vi "CO2FeedbackControl.vi"() -> ()   [LabVIEW 2020]
uses:
  <vilib>/Utility/file.llb/Write Delimited Spreadsheet (DBL).vi
  <vilib>/Analysis/NI_AALPro.lvlib
panel:
  in  "N":i32=30
  in  "file path (dialog if empty) 3":path=path "C:/Users/user/Desktop/CO2_Laptop/Data/data"
  in  "format (%.3f) 2":string="%.5f"
  in  "Save File 2":bool
  in  "file path (dialog if empty) 4":path=path "C:/Users/user/Desktop/CO2_Laptop/Data/210528"
  out "appended path 3":path=path "C:/Users/user/Desktop/CO2_Laptop/Data/210528/81757"
  in  "Save All":bool
  in  "Saving File Time(Sec)":dbl=60.0
  in  "Safty Check":bool=TRUE
  out "> Thres 2":bool
  in  "Slope Set":dbl=300.0
  out "Time Number":u32=81757
  out "String":string="081757\r\n"
  in  "Save Background":bool
  out "> Thres":bool
  in  "stop":bool
  in  "Integration Time(ms)":i32=85
  in  "Average Times":i32=4
  in  "Wait Time":u32=120
  in  "UV450 Set":sgl=383500.0
  in  "Rate (ml/min)":dbl=0.0045
  out "Dose or Not":i32
  in  "Pump Time":u32=1000
  in  "Connect the Pump":bool=TRUE
  in  "Setting Tab":T1(tab)
  out "On/Off":i32(graph)
  out "Derative Signal":dbl(graph)=-0.9345383759733037
  out "FADH":sgl(graph)=81856.375
  out "?":sgl=81856.375
  out "?":sgl=1683298.0
  out "UV300":sgl=1683274.0
  out "Fc+":sgl(graph)=1683274.0
  out "NADH":sgl(graph)=1683298.0
  out "U300 Slope":dbl=-0.9345383759733037
  in  "Initial Number":dbl
  in  "Initial Wavelength 2":dbl=275.0
  out "Index 2":dbl=125.0
  in  "Final Wavelength":dbl=620.0
  out "Index 3":dbl=576.0
  out "subarray 2":sgl[](array[numeric])=[332.8669, 333.6288, 334.39072, 335.15262, 335.9145, 336.67633, 337.43814, 338.19995, 338.96173, 339.72348, 340.4852, 341.24692, 342.0086, 342.77026, 343.53192, 344.29355, 345.05515, 345.8167, 346.57825, 347.33978, 348.10126, 348.86273, 349.6242, 350.38562, 351.147, 351.9084]
  out "subarray":sgl[](array[numeric])=[446.05103, 446.80762, 447.56418, 448.32068, 449.07715, 449.83356, 450.5899, 451.34622, 452.1025, 452.8587, 453.6149, 454.371, 455.12708, 455.8831, 456.63907, 457.395, 458.15088, 458.9067, 459.66248, 460.4182, 461.1739, 461.92953, 462.68512, 463.44064, 464.19614, 464.95157]
  in  "index":i32=350
  in  "length 3":i32=26
  in  "index 2":i32=201
  out "Background":sgl[](graph)=[172.21637, 178.6098, 190.38326, 201.36111, 203.4611, 197.77924, 190.34503, 202.32442, 224.52594, 247.76048, 288.25705, 329.7657, 369.02264, 416.01242, 476.80292, 575.00824, 737.26373, 961.8769, 1266.476, 1647.3512, 2141.3354, 2791.3042, 3647.9653, 4759.415, 6167.531, 7863.0625, 9861.403, 12171.496, 14761.8125, 17573.484, 20526.473, 23478.443, 26351.168, 29083.691, 31614.525, 33886.91, 35870.95, 37502.207, 38754.105, 39600.734, 40049.812, 40105.33, 39828.324, 39231.23, 38360.957, 37355.445, 36104.72, 34783.223, 33399.88, 31985.346, 30560.78, 29142.305, 27749.982, 26391.615, 25085.277, 23821.594, 22594.584, 21429.28, 20331.139, 19246.326, 18235.92, 17305.72, 16387.797, 15554.422, 14779.023, 14065.231, 13400.149, 12777.7295, 12199.317, 11662.219, 11158.4375, 10707.728, 10302.769, 9948.339, 9619.979, 9311.22, 9019.734, 8746.263, 8497.579, 8287.871, 8119.847, 7988.0596, 7882.8696, 7806.2563, 7740.983, 7700.281, 7682.2935, 7665.853, 7679.71, 7699.8457, 7742.342, 7819.9507, 7932.1553, 8081.9766, 8245.204, 8436.354, 8637.018, 8861.075, 9118.328, 9391.317, 9705.655, 10059.682, 10457.724, 10911.704, 11425.339, 11995.643, 12610.294, 13264.511, 13950.56, 14684.349, 15458.021, 16279.438, 17157.658, 18103.229, 19112.172, 20207.807, 21388.975, 22639.855, 23991.432, 25457.422, 27022.8, 28664.277, 30323.066, 32030.035, 33610.438, 35245.04, 36934.887, 38771.98, 40825.938, 43076.9, 45512.37, 48168.47, 50984.766, 53626.605, 56118.92, 58950.207, 61775.047, 63773.973, 63949.07, 64084.047, 64178.383, 64184.605, 64149.074, 64052.793, 63915.992, 63918.89, 64040.336, 64118.902, 64116.21, 64092.902, 64052.22, 64033.504, 64038.297, 64028.242, 64027.098, 64060.793, 64076.066, 64126.375, 64043.8, 63250.496, 61768.496, 60734.766, 59729.53, 57698.125, 54165.81, 50176.914, 46149.234, 42733.66, 39790.543, 37493.91, 35500.812, 33451.094, 31229.004, 28788.117, 26540.094, 24475.693, 22718.572, 21113.527, 19627.281, 18206.932, 16862.273, 15712.507, 14730.38, 13751.289, 12770.087, 11858.61, 11046.73, 10340.737, 9747.756, 9237.91, 8805.616, 8444.61, 8120.295, 7834.2686, 7539.886, 7164.0596, 6707.6084, 6190.263, 5689.185, 5312.52, 5098.453, 4977.2, 4910.097, 4891.2104, 4864.877, 4698.309, 4427.4155, 4232.314, 4121.4736, 4006.222, 3878.76, 3771.4011, 3690.84, 3640.2373, 3603.596, 3591.162, 3573.36, 3571.922, 3578.0845, 3617.4995, 3670.426, 3743.4565, 3818.7466, 3857.2388, 3859.1992, 3828.7473, 3787.6472, 3752.0144, 3739.1199, 3729.3882, 3729.4111, 3711.954, 3675.612, 3636.6428, 3600.4456, 3568.309, 3558.572, 3548.6543, 3553.8538, 3585.2307, 3649.1536, 3724.6, 3798.702, 3789.903, 3713.3398, 3570.3772, 3424.1174, 3351.6611, 3369.2878, 3452.262, 3535.7366, 3538.5234, 3437.643, 3262.2917, 3037.4912, 2832.5955, 2661.3347, 2508.405, 2392.6135, 2306.7063, 2273.7944, 2276.2817, 2301.8428, 2296.0056, 2258.3638, 2196.5005, 2115.8386, 2057.6409, 2045.1534, 2070.7346, 2122.393, 2100.536, 2018.3241, 1882.6237, 1799.5573, 1897.3712, 2203.182, 2784.7966, 3397.9448, 3467.0032, 2968.6287, 2293.2832, 1670.7052, 1317.4867, 1272.086, 1250.7498, 1187.051, 1207.0577, 1242.5907, 1185.1292, 1063.2871, 986.917, 961.3804, 934.924, 907.7848, 873.4408, 833.07916, 792.1351, 748.04736, 694.6823, 654.212, 617.8926, 585.5748, 555.31824, 530.2687, 512.13306, 502.65018, 484.0129, 461.54538, 436.27756, 404.15952, 379.0401, 336.2221, 303.73672, 269.4475, 242.80533, 231.45448, 222.27428, 226.29994, 221.17111, 211.7707, 199.02214, 187.00967, 167.50746, 160.57787, 158.06314, 145.95668, 140.2896, 143.32124, 142.59326, 145.61113, 140.5319, 125.95628, 115.798744, 104.68489, 91.8871, 84.10792, 83.73946, 79.02437, 89.39399, 93.75515, 103.549706, 113.17898, 119.95357, 112.730675, 107.5902, 98.01945, 93.53506, 81.586525, 71.61932, 63.659184, 70.39902, 75.41178, 91.91837, 104.64616, 116.470856, 121.41953, 125.59211, 116.32846, 110.59207, 97.97765, 85.71354, 72.04285, 70.710396, 77.94153, 104.69237, 128.20029, 134.88873, 131.4962, 110.10464, 84.07277, 67.67252, 59.044857, 58.778107, 64.593765, 69.131714, 66.15145, 69.076164, 71.793076, 71.89148, 69.14369, 61.262066, 54.19736, 46.46217, 35.316803, 10.673843, 0.65000325, 3.4500182, 21.898348, 51.27786, 87.18853, 101.60523, 93.91958, 76.44091, 50.19149, 32.17609, 34.534836, 40.355633, 55.11234, 64.29569, 72.62746, 80.33474, 80.12523, 75.10533, 67.51369, 49.410484, 36.219204, 26.42124, 36.805626, 43.322285, 58.033817, 65.59648, 68.226845, 64.07072, 62.22196, 56.900043, 44.901432, 42.843807, 33.538353, 31.444857, 31.923042, 27.305967, 28.892494, 34.93258, 44.089443, 56.331985, 72.50936, 71.152855, 65.88946, 58.713154, 44.860325, 35.122955, 25.37532, 20.282688, 20.226677, 29.445103, 47.947227, 68.52041, 90.17749, 103.97235, 99.2943, 81.80186, 61.792732, 48.94577, 34.207508, 40.06172, 48.37855, 54.032833, 64.7118, 79.192184, 89.2192, 95.4683]
  in  "index 3":i32=145
  in  "length":i32=26
  out "subarray 3":sgl[](array[numeric])=[290.1744, 290.93707, 291.6997, 292.46237, 293.225, 293.98764, 294.75027, 295.5129, 296.2755, 297.03812, 297.80072, 298.56332, 299.3259, 300.08847, 300.851, 301.6136, 302.37613, 303.13864, 303.90118, 304.6637, 305.42618, 306.1887, 306.95117, 307.71362, 308.47607, 309.23853]
  out "While Number Now":dbl=60.0
  in  "Wavelength":dbl=455.0
  out "Index":dbl=360.0
  in  "Slope":bool=TRUE
  out "subarray 5":dbl[](array[numeric])=[1683269.0, 1683298.375, 1683359.625, 1683206.625, 1683395.5, 1683321.875, 1683329.125, 1683184.25, 1683210.75, 1683321.25, 1683323.75, 1683204.75, 1683348.5, 1683351.75, 1683382.25, 1683268.0, 1683432.25, 1683458.25, 1683313.375, 1683185.25, 1683231.25, 1683440.875, 1683121.25, 1683666.5, 1683304.0, 1683178.75, 1683377.75, 1683289.5, 1683221.625, 1683048.25]
  out "Array 2":i32[](array[numeric])=[1, 2, 3, 4, 5, 6, 7, 8, 9, 10, 11, 12, 13, 14, 15, 16, 17, 18, 19, 20, 21, 22, 23, 24, 25, 26, 27, 28, 29, 30]
  out "Raw Data Graph 3":cluster{"Lumda":sgl[], "Intensity":sgl[]}(graph)
  out "Trans (Signal >275nm is more stable)":cluster{"Lumda":sgl[], "Intensity":sgl[]}(graph)
  # "Signal Up; More Transparent"
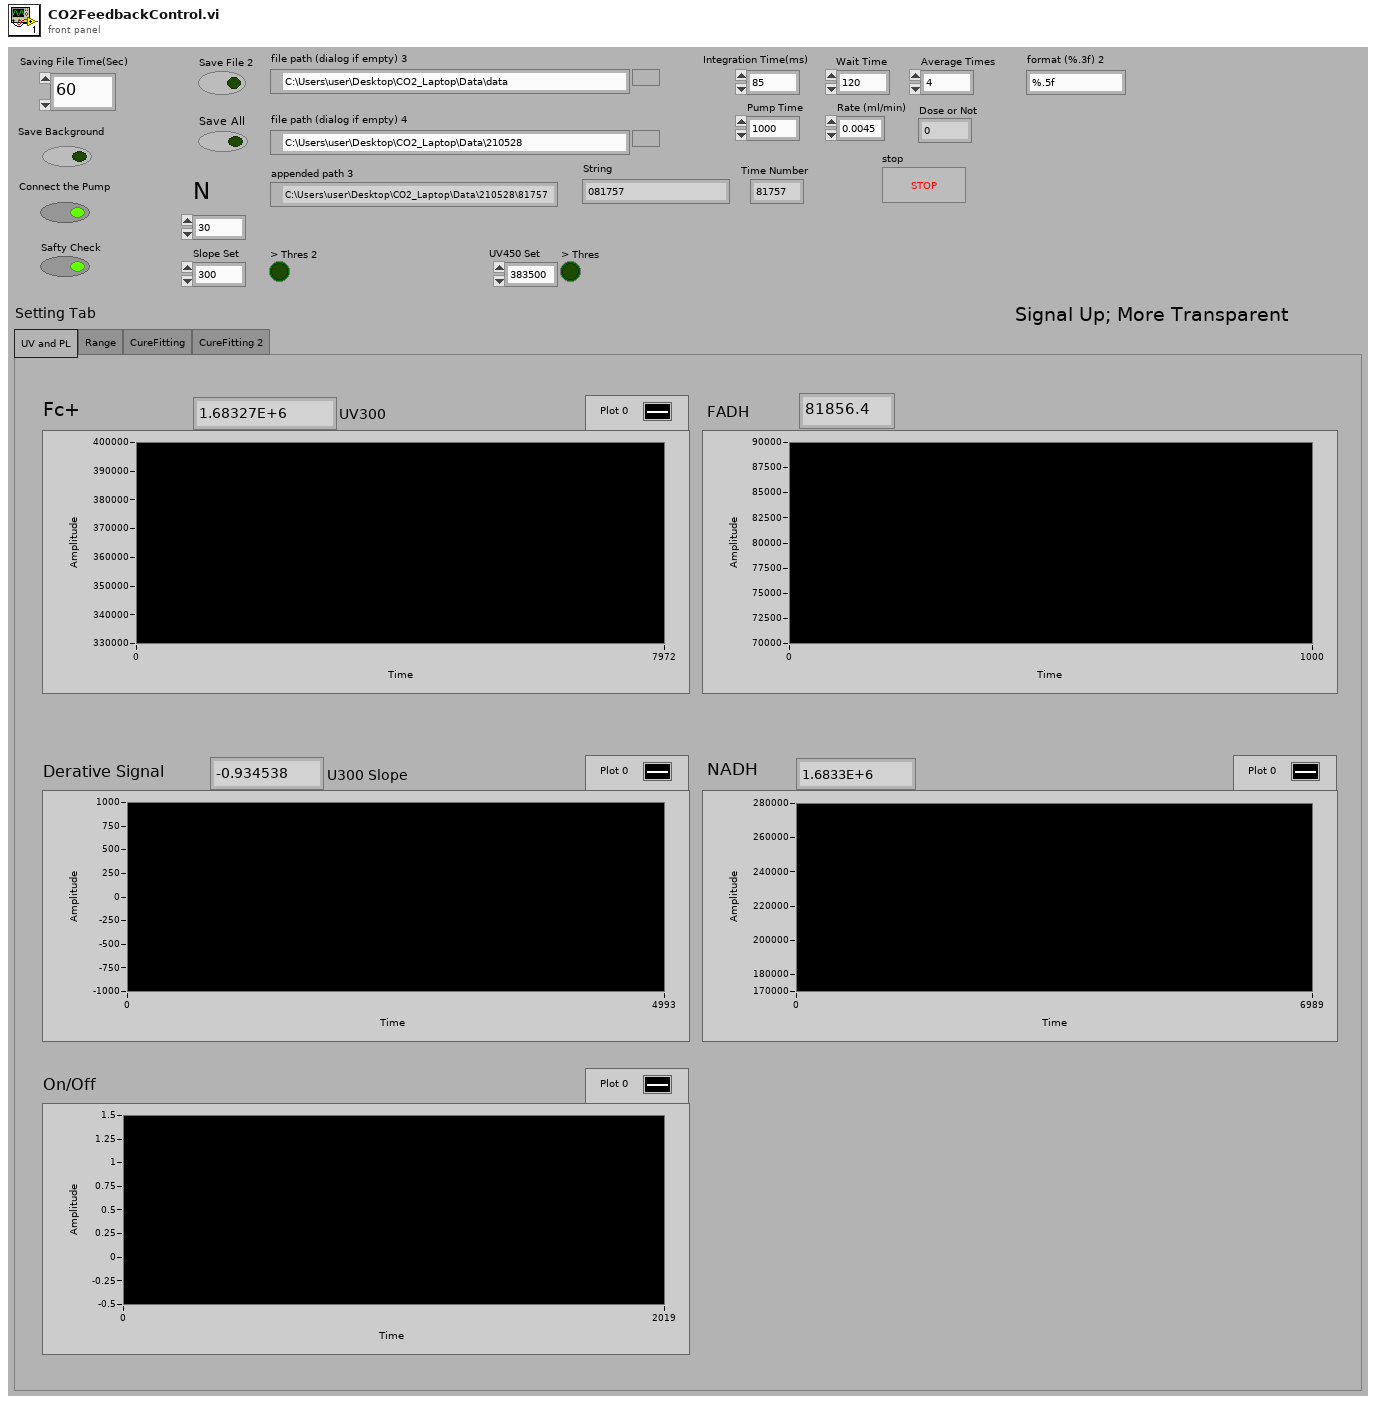
[diagram p1: front panel]
types:
  T1 = enum32{"UV and PL", "Range", "CureFitting", "CureFitting 2"}
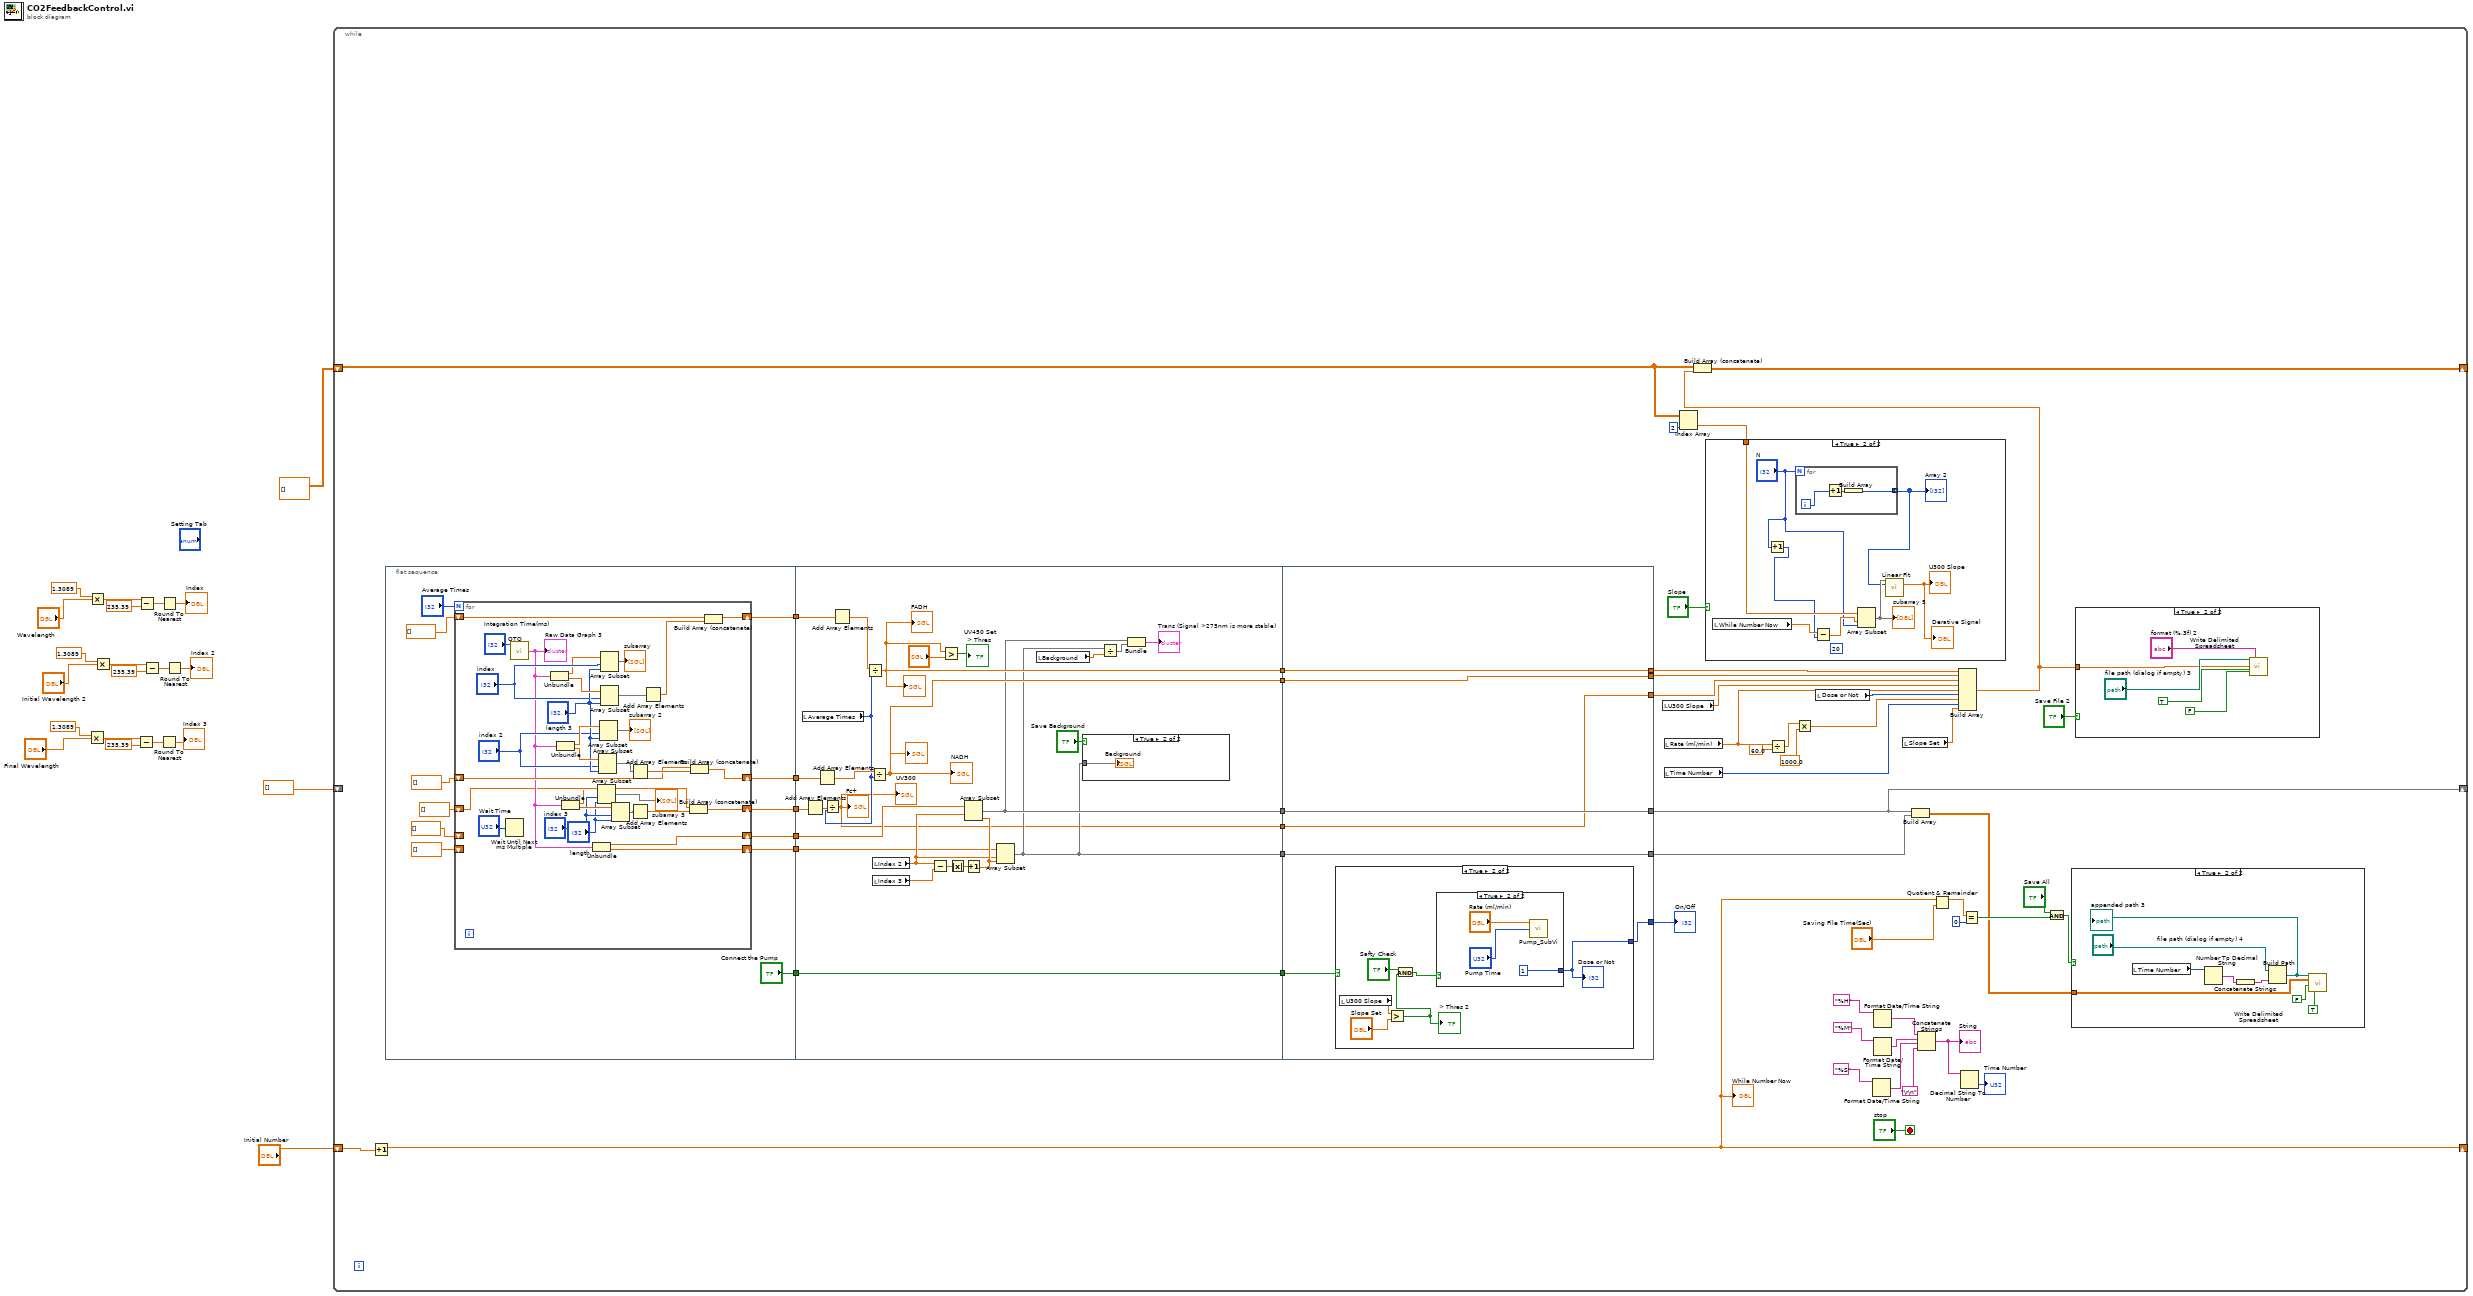
[diagram p0: block diagram]
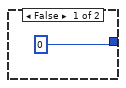
[diagram p6: hidden frame]
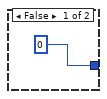
[diagram p7: hidden frame]
diagram:
  n1 = Multiply(x=1.3089, y="Final Wavelength") -> (x*y=w7:dbl)
  n2 = Multiply(x=1.3089, y="Wavelength") -> (x*y=w20:dbl)
  n3 = Multiply(x=1.3089, y="Initial Wavelength 2") -> (x*y=w13:dbl)
  n4 = Subtract(x=w7, y=235.39) -> (x-y=w6:dbl)
  n5 = Subtract(x=w20, y=235.39) -> (x-y=w19:dbl)
  n6 = Subtract(x=w13, y=235.39) -> (x-y=w12:dbl)
  n7 = Round To Nearest(number=w6) -> (nearest integer value=→"Index 3":dbl)
  n8 = Round To Nearest(number=w19) -> (nearest integer value=→"Index":dbl)
  n9 = Round To Nearest(number=w12) -> (nearest integer value=→"Index 2":dbl)
  n10 = while {
    shift-right: [w67] -> _
    shift-left: sgl[][] [] -> [w48]
    shift-right: [w30] -> _
    shift-left: sgl[] [] -> [_]
    shift-right: [w23] -> _
    shift-left: "Initial Number" -> [w49]
    stop <- "stop" stop-if-true
    n11 = Increment(x=w49) -> (x+1=w23:dbl)
    "While Number Now" <- w23
    n12 = flat-sequence {
      tunnel: [w105] -> w73
      tunnel: [w104] -> w72
      tunnel: ["Connect the Pump"] -> w68
      tunnel: [w102] -> w66
      tunnel: [w101] -> w65
      tunnel: [w99] -> w52
      tunnel: w73 -> [w156]
      tunnel: w72 -> [w155]
      tunnel: [w158] -> w71
      tunnel: [w157] -> w70
      tunnel: [w154] -> w69
      tunnel: w68 -> [w154]
      tunnel: w66 -> [w153]
      tunnel: w65 -> [w152]
      tunnel: [w147] -> w63
      tunnel: [w149] -> w62
      tunnel: w52 -> [w145]
      tunnel: [w142] -> w51
      tunnel: [w174] -> w26
      tunnel: [w175] -> w27
      tunnel: w71 -> [w175]
      tunnel: w70 -> [w174]
      tunnel: w69 -> [w173]
      tunnel: [w172] -> w64
      tunnel: w63 -> [w172]
      tunnel: w62 -> [w171]
      tunnel: [w171] -> w30
      tunnel: w51 -> [w170]
      tunnel: [w170] -> w28
      tunnel: [w169] -> w22
      frame #0 {
        n13 = for {
          N: "Average Times" -> [_]
          shift-right: [w135] -> w105
          shift-left: sgl[] [] -> [w134]
          shift-right: [w131] -> w104
          shift-left: sgl[] [] -> [w130]
          shift-right: [w127] -> w101
          shift-left: sgl[] [] ("Intensity") -> [_]
          shift-right: [w126] -> w102
          shift-left: sgl[] [] -> [_]
          shift-right: [w116] -> w99
          shift-left: sgl[] [] -> [w115]
          n14 = Wait Until Next ms Multiple(millisecond multiple="Wait Time") -> ()  [unwired: 1 out]
          n15 = call "OTO.vi"("Integration Time(ms)"="Integration Time(ms)") -> ("Raw Data Graph"=w119:cluster{"Lumda":sgl[], "Intensity":sgl[]})  [unwired: 2 in]
          "Raw Data Graph 3" <- w119
          n16 = Unbundle(w119) -> ("Lumda"=w123:sgl[], "Intensity"=w140:sgl[])
          n17 = Unbundle(w119) -> ("Lumda"=w139:sgl[], "Intensity"=w138:sgl[])
          n18 = Unbundle(w119) -> ("Lumda"=w113:sgl[], "Intensity"=w118:sgl[])
          n19 = Unbundle(w119) -> ("Lumda"=w126:sgl[], "Intensity"=w127:sgl[])
          n20 = Array Subset(array=w113, index="index 3", length="length") -> (→"subarray 3":sgl[])
          n21 = Array Subset(array=w138, index="index 2", length="length 3") -> (w128:sgl[])
          n22 = Array Subset(array=w139, index="index 2", length="length 3") -> (→"subarray 2":sgl[])
          n23 = Array Subset(array=w140, index="index", length="length 3") -> (w133:sgl[])
          n24 = Array Subset(array=w123, index="index", length="length 3") -> (→"subarray":sgl[])
          n25 = Array Subset(array=w118, index="index 3", length="length") -> (w120:sgl[])
          n26 = Add Array Elements(numeric array=w128) -> (sum=w132:sgl)
          n27 = Add Array Elements(numeric array=w120) -> (sum=w117:sgl)
          n28 = Add Array Elements(numeric array=w133) -> (sum=w129:sgl)
          n29 = Build Array (concatenate)(w115, w117) -> (w116:sgl[])
          n30 = Build Array (concatenate)(w130, w132) -> (w131:sgl[])
          n31 = Build Array (concatenate)(w134, w129) -> (w135:sgl[])
        }
      }
      frame #1 {
        n32 = local read "Average Times"() -> (w143:i32)
        n33 = Add Array Elements(numeric array=w145) -> (sum=w144:sgl)
        n34 = Add Array Elements(numeric array=w155) -> (sum=w159:sgl)
        n35 = Divide(x=w144, y=w143) -> (x/y=w142:sgl)
        "Fc+" <- w142
        "UV300" <- w142
        n36 = Add Array Elements(numeric array=w156) -> (sum=w160:sgl)
        n37 = Divide(x=w160, y=w143) -> (x/y=w157:sgl)
        "FADH" <- w157
        "?" <- w157
        n38 = Divide(x=w159, y=w143) -> (x/y=w158:sgl)
        "NADH" <- w158
        "?" <- w158
        n39 = local read "Index 2"() -> (w166:dbl)
        n40 = local read "Index 3"() -> (w163:dbl)
        n41 = Subtract(x=w166, y=w163) -> (x-y=w162:dbl)
        n42 = Greater?(x=w157, y="UV450 Set") -> (0:→"> Thres":bool)
        n43 = Absolute Value(x=w162) -> (abs(x)=w161:dbl)
        n44 = Increment(x=w161) -> (x+1=w167:dbl)
        n45 = Array Subset(array=w153, index=w166, length=w167) -> (w149:sgl[])
        n46 = Array Subset(array=w152, index=w166, length=w167) -> (w147:sgl[])
        n47 = local read "Background"() -> (w148:sgl[])
        n48 = case shown="True" "Save Background" {
          tunnel: w147 -> [_ w168]
          frame False {
          }
          frame True {
            "Background" <- w168
          }
        }
        n49 = Divide(x=w147, y=w148) -> (x/y=w146:sgl[])
        n50 = Bundle(w149, w146) -> (→"Trans (Signal >275nm is more stable)":cluster{sgl[], sgl[]})  [unwired: 1 in]
      }
      frame #2 {
        n51 = case shown="True" w173 {
          tunnel: [0 w177] -> w169
          frame False {
          }
          frame True {
            n52 = local read "U300 Slope"() -> (w182:dbl)
            n53 = Greater?(x=w182, y="Slope Set") -> (0:w180:bool)
            "> Thres 2" <- w180
            n54 = And(x="Safty Check", y=w180) -> (x .and. y?=w179:bool)
            n55 = case shown="True" w179 {
              tunnel: [0 1] -> w177
              frame False {
              }
              frame True {
                n56 = call "Pump_SubVi.vi"("Each Pumping Time"="Pump Time", "rate (ml/min)"="Rate (ml/min)") -> ()  [unwired: 1 in]
              }
            }
            "Dose or Not" <- w177
          }
        }
      }
    }
    n57 = local read "U300 Slope"() -> (w25:dbl)
    n58 = local read "Rate (ml/min)"() -> (w44:dbl)
    n59 = local read "Time Number"() -> (w39:u32)
    n60 = Index Array(array=w48, index (col)=2 ("index (row)")) -> (element=w46:dbl[])  [unwired: 1 in]
    n61 = case shown="True" "Slope" {
      tunnel: w46 -> [_ w95]
      frame False {
      }
      frame True {
        (unwired) 20 ("length")
        n62 = local read "While Number Now"() -> (w94:dbl)
        n63 = Increment(x="N") -> (x+1=w89:i32)
        n64 = for {
          N: "N" -> [_]
          tunnel: [w96] -> w90 mode=concatenating
          i -> [w97]
          n65 = Increment(x=w97) -> (x+1=w98:i32)
          n66 = Build Array(w98) -> (w96:i32[])
        }
        "Array 2" <- w90
        n67 = Subtract(x=w94, y=w89) -> (x-y=w93:dbl)
        n68 = Array Subset(array=w95, index=w93, length="N") -> (w92:dbl[])
        "subarray 5" <- w92
        n69 = call <vilib>:"Linear Fit.vi"("Y"=w92, "X"=w90) -> ("slope"=→"U300 Slope" →"Derative Signal":dbl)  [unwired: 9 in, 4 out]
      }
    }
    n70 = Divide(x=w44, y=60.0) -> (x/y=w42:dbl)
    n71 = Multiply(x=w42, y=1000.0) -> (x*y=w40:dbl)
    n72 = local read "Dose or Not"() -> (w45:i32)
    n73 = Format Date/Time String(time format string (%c)="%S") -> (date/time string=w56:string)  [unwired: 2 in]
    n74 = Format Date/Time String(time format string (%c)="%H") -> (date/time string=w58:string)  [unwired: 2 in]
    n75 = Format Date/Time String(time format string (%c)="%M") -> (date/time string=w57:string)  [unwired: 2 in]
    n76 = local read "Slope Set"() -> (w38:dbl)
    n77 = Build Array(w30, w64) -> (w31:sgl[][])
    n78 = Concatenate Strings(w58, w57, w56, "\r\n") -> (w54:string)
    "String" <- w54
    n79 = Quotient & Remainder(x=w23, y="Saving File Time(Sec)") -> (x-y*floor(x/y)=w35:dbl)  [unwired: 1 out]
    n80 = Build Array(w26, w27, w28, w25, w44, w45, w40, w39, w38) -> (w24:dbl[])
    n81 = Build Array (concatenate)(w48, w24) -> (w67:dbl[][])
    n82 = Decimal String To Number(string=w54) -> (number=→"Time Number":i32)  [unwired: 2 in, 1 out]
    n83 = Equal?(x=w35, y=0) -> (x = y?=w36:bool)
    n84 = And(x="Save All", y=w36) -> (x .and. y?=w33:bool)
    n85 = case shown="True" w33 {
      tunnel: w31 -> [_ w82]
      frame False {
      }
      frame True {
        n86 = local read "Time Number"() -> (w80:u32)
        n87 = Number To Decimal String(number=w80) -> (decimal integer string=w81:string)  [unwired: 1 in]
        n88 = Concatenate Strings(w81) -> (w87:string)
        n89 = Build Path(base path="file path (dialog if empty) 4", name or relative path=w87) -> (appended path=w86:path)
        "appended path 3" <- w86
        n90 = call-poly <vilib>:"Write Delimited Spreadsheet.vi"("file path (dialog if empty)"=w86, "2D data"=w82, "append to file? (new file:F)"=FALSE ("transpose? (no:F)"), "transpose? (no:F)"=TRUE) -> ()  [unwired: 10 in, 2 out]
      }
    }
    n91 = case shown="True" "Save File 2" {
      tunnel: w24 -> [_ w76]
      frame False {
      }
      frame True {
        n92 = call-poly <vilib>:"Write Delimited Spreadsheet.vi"("file path (dialog if empty)"="file path (dialog if empty) 3", "format (%.3f)"="format (%.3f) 2", "1D data"=w76, "append to file? (new file:F)"=TRUE, "transpose? (no:F)"=FALSE) -> ()  [unwired: 9 in, 2 out]
      }
    }
    "On/Off" <- w22
  }
